vi "CRYAna Broadband RMS.vi"(8 "Info":T1={"Fs"=44100.0, "discard cycles"=3.0, "Sens In"=0.0, "AC/DC"=0} {"Fs" min=1.0; "Sens In" format="%.2f"; "discard cycles" min=1.0}, 9 "Freq":dbl[](array[numeric]), 10 "Cycles":dbl[](array[numeric]), 11 "Response":dbl[](array[numeric])) -> (3 "Freq resp curves":cluster{cluster{"Fi":dbl, dbl, dbl}[]}[](array[cluster]))   [LabVIEW 2013]
uses:
  <vilib>/Analysis/NI_AALPro.lvlib
panel:
  out "XY Graph":cluster{cluster{"Fi":dbl, dbl}[]}[](graph)
  # "Broadband RMS"
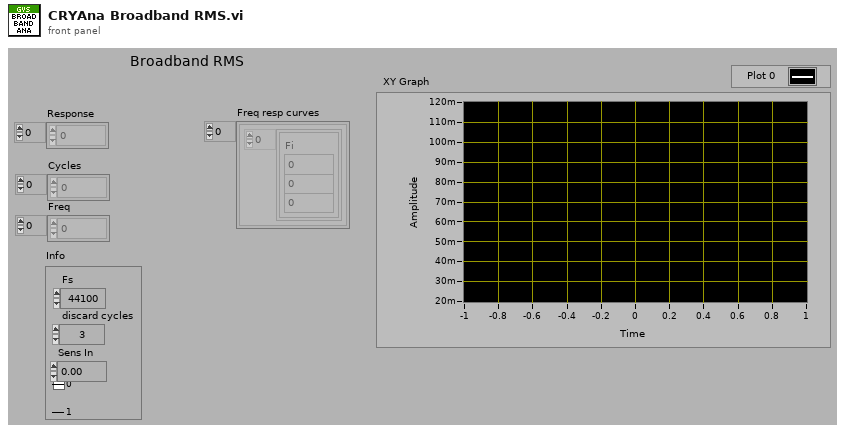
[diagram p1: front panel]
types:
  T1 = cluster{"Fs":dbl, "discard cycles":dbl, "Sens In":dbl, "AC/DC":i32}
  T2 = cluster{"Fi":dbl, "DC estimate (V)":dbl, "DC estimate (V)":dbl}[]
  T3 = cluster{cluster{"Fi":dbl, "DC estimate (V)":dbl, "DC estimate (V)":dbl}[]}
  T4 = cluster{cluster{"Fi":dbl, "DC estimate (V)":dbl}[]}
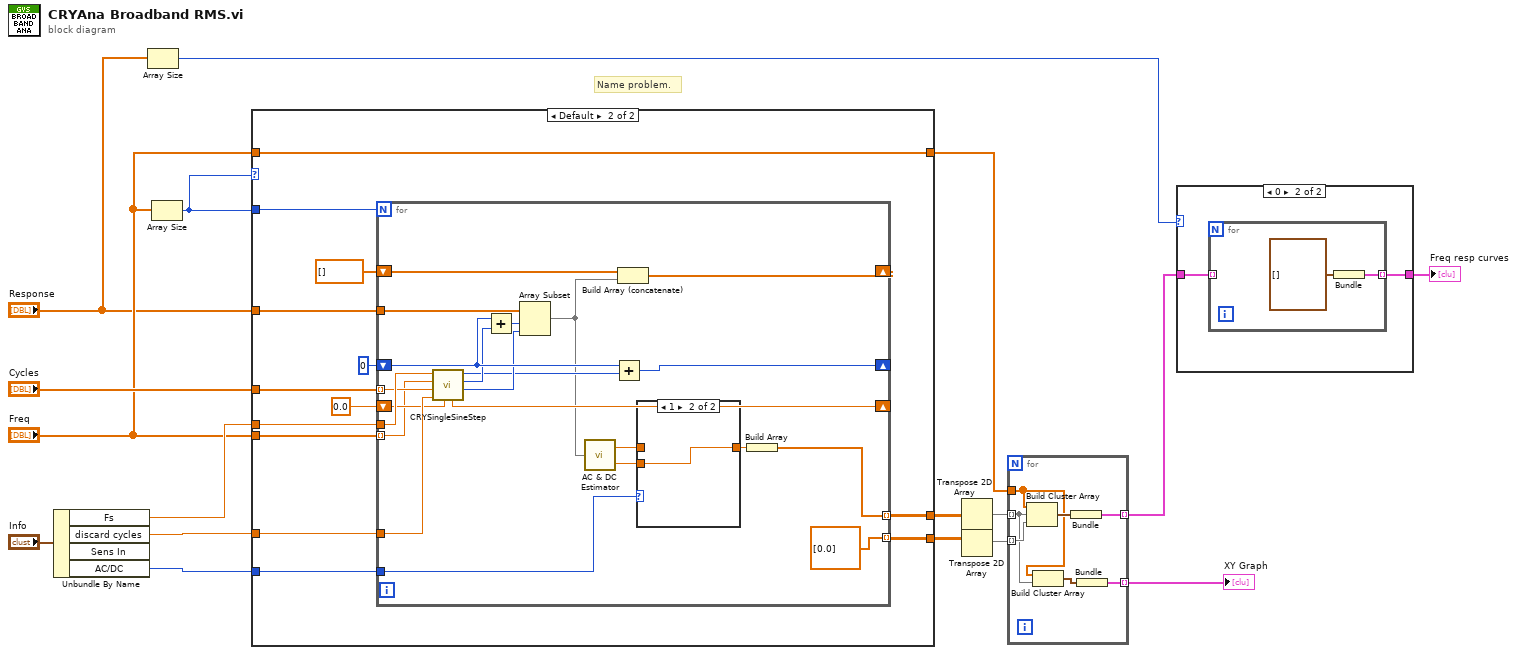
[diagram p0: block diagram]
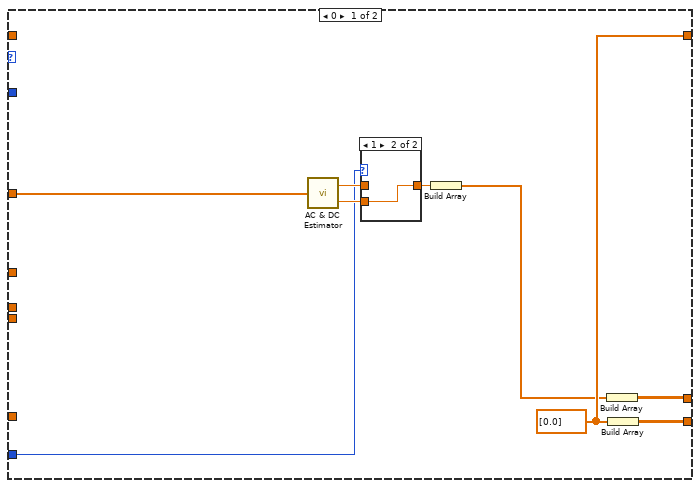
[diagram p3: hidden frame]
diagram:
  # "Name problem."
  n1 = Unbundle By Name("Info") -> ("Fs"=w10:dbl, "discard cycles"=w9:dbl, "AC/DC"=w11:i32)  [unwired: 1 out]
  n2 = Array Size(array="Response") -> (size(s)=w3:i32)
  n3 = Array Size(array="Freq") -> (size(s)=w8:i32)
  n4 = case shown="Default" w8 {
    tunnel: w8 -> [_ w39]
    tunnel: [w21 w38] -> w17
    tunnel: [w20 w37] -> w16
    tunnel: "Response" -> [w22 w35]
    tunnel: "Freq" -> [_ w34]
    tunnel: "Cycles" -> [_ w33]
    tunnel: w11 -> [w23 w32]
    tunnel: w10 -> [_ w31]
    tunnel: w9 -> [_ w30]
    tunnel: "Freq" -> [_ w29]
    tunnel: [w19 w29] -> w6
    frame 0 {
      w19 = dbl[] [0.0]
      n5 = call <vilib>:"AC & DC Estimator.vi"("Signal (V)"=w22) -> ("AC estimate (Vrms)"=w26:dbl, "DC estimate (V)"=w25:dbl)
      n6 = case shown="1" w23 {
        tunnel: w26 -> [w27 _]
        tunnel: w25 -> [_ w28]
        tunnel: [w27 w28] -> w24
        frame 0, Default {
        }
        frame 1 {
        }
      }
      n7 = Build Array(w24) -> (w18:dbl[])
      n8 = Build Array(w18) -> (w21:dbl[][])
      n9 = Build Array(w19) -> (w20:dbl[][])
    }
    frame Default {
      n10 = for {
        N: w39 -> [_]
        tunnel: w31 -> [w58]
        shift-right: [w61] -> _
        shift-left: 0 -> [w59]
        tunnel: w35 -> [w62]
        shift-right: [w63] -> _
        shift-left: dbl[] [] -> [w50]
        tunnel: w33 -> [w57] mode=indexing
        tunnel: w34 -> [w52] mode=indexing
        tunnel: [w42] -> w38 mode=indexing
        tunnel: [dbl[] [0.0]] -> w37 mode=indexing
        tunnel: w30 -> [w56]
        shift-right: [w49] -> _
        shift-left: 0.0 -> [w53]
        tunnel: w32 -> [w44]
        n11 = call "CRYSingleSineStep.vi"("Fs"=w58, "Freq"=w52, "Cycles per freq"=w57, "Cycles discarded"=w56, "StartPhase"=w53) -> ("StopPhase"=w49:dbl, "TotalSamples"=w51:i32, "DiscardSamples"=w54:i32, "ExtractSamples"=w55:i32)  [unwired: 2 out]
        n12 = Add(x=w59, y=w54) -> (x+y=w60:i32)
        n13 = Array Subset(array=w62, index=w60, length=w55) -> (w48:dbl[])
        n14 = call <vilib>:"AC & DC Estimator.vi"("Signal (V)"=w48) -> ("AC estimate (Vrms)"=w47:dbl, "DC estimate (V)"=w46:dbl)
        n15 = Add(x=w59, y=w51) -> (x+y=w61:i32)
        n16 = Build Array (concatenate)(w50, w48) -> (w63:dbl[])
        n17 = case shown="1" w44 {
          tunnel: w47 -> [w64 _]
          tunnel: w46 -> [_ w65]
          tunnel: [w64 w65] -> w45
          frame 0, Default {
          }
          frame 1 {
          }
        }
        n18 = Build Array(w45) -> (w42:dbl[])
      }
    }
  }
  n19 = Transpose 2D Array(2D array=w17) -> (transposed array=w15:dbl[][])
  n20 = Transpose 2D Array(2D array=w16) -> (transposed array=w14:dbl[][])
  n21 = for {
    tunnel: w15 -> [w67] mode=indexing
    tunnel: w14 -> [w72] mode=indexing
    tunnel: w6 -> [w68]
    tunnel: [w70] -> w2 mode=indexing
    tunnel: [w66] -> w5 mode=indexing
    n22 = Build Cluster Array(w68, w67, w72) -> (w71:T2)
    n23 = Build Cluster Array(w68, w67) -> (w69:cluster{"Fi":dbl, "DC estimate (V)":dbl}[])
    n24 = Bundle(w71) -> (w70:T3)  [unwired: 1 in]
    n25 = Bundle(w69) -> (w66:T4)  [unwired: 1 in]
  }
  "XY Graph" <- w5
  n26 = case shown="0" w3 {
    tunnel: w2 -> [w73 w75]
    tunnel: [w73 w74] -> w1
    frame 1, Default {
    }
    frame 0 {
      n27 = for {
        tunnel: w75 -> [_] mode=indexing
        tunnel: [w76] -> w74 mode=indexing
        n28 = Bundle(T2 []) -> (w76:T3)  [unwired: 1 in]
      }
    }
  }
  "Freq resp curves" <- w1
